vi "EG_G5210 VisaRW.vi"(0 "VISA Rsrc":refnum<visa-resource-name>="GPIB0::12::INSTR", 1 "EOS (Aucun)":string, 5 "ChaineCom":string caption="Chaîne de commande", 6 "Délais (0 ms)":u32, 7 "LockIfc":bool, 9 "Nbcaract":u32=100 caption="Nombre de \ncaractères à lire", 11 "error in (no error)":errorcluster, 12 "Lecture?(T)":bool=TRUE, 13 "Timeout(ms)":u32=2000) -> (4 "VISA Rsrc Out":refnum<visa-resource-name>="GPIB0::12::INSTR", 10 "ChaineRep":string caption="Chaîne de réponse", 14 "Count out":u32=44 caption="Nombre de caractères lus", 15 "error out":errorcluster)   [LabVIEW 2019]
doc: "Ce VI envoie des commande d'écriture et de lecture VISA à l'appareil GPIB. Il permet de ne pas séparer un question de sa réponse. Pour que cela fonctionne toute lecture d'un instrument doit se faire par ce VI."
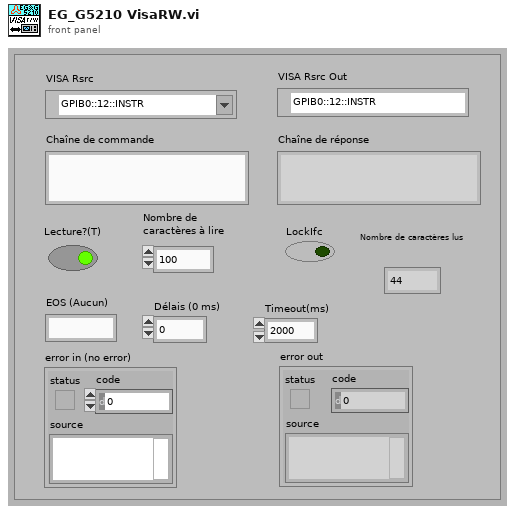
[diagram p1: front panel]
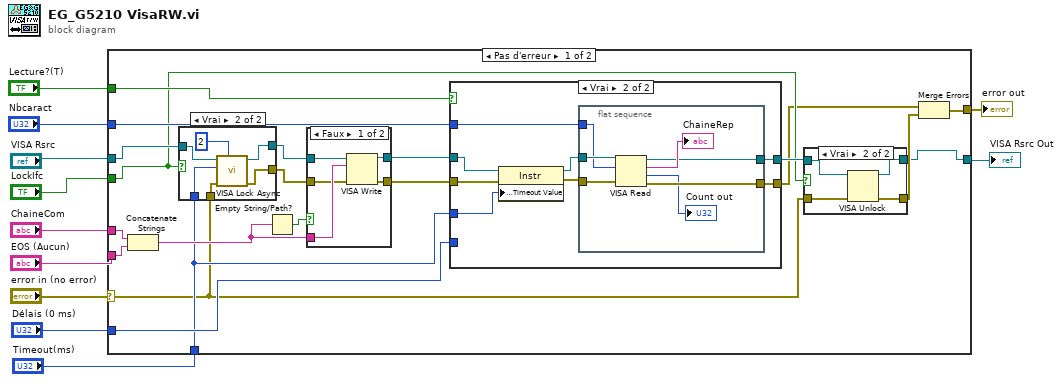
[diagram p0: block diagram]
diagram:
  n1 = case shown="Pas d'erreur" "error in (no error)" {
    selector: "error in (no error)" -> [w16 w71]
    tunnel: "VISA Rsrc" -> [w22 w70]
    tunnel: [w12 w70] -> w3
    tunnel: "ChaineCom" -> [w31 _]
    tunnel: "EOS (Aucun)" -> [w30 _]
    tunnel: "Délais (0 ms)" -> [w27 _]
    tunnel: "Nbcaract" -> [w26 _]
    tunnel: "Lecture?(T)" -> [w25 _]
    tunnel: [w14 w71] -> w5
    tunnel: "Timeout(ms)" -> [w17 _]
    tunnel: "LockIfc" -> [w18 _]
    frame No Error {
      n2 = Concatenate Strings(w31, w30) -> (w23:string)
      n3 = case shown="Vrai" w18 {
        tunnel: [w38 w45] -> w20
        tunnel: w16 -> [w38 w44]
        tunnel: w22 -> [w39 w43]
        tunnel: w17 -> [_ w42]
        tunnel: [w39 w41] -> w21
        frame False {
        }
        frame True {
          n4 = call <vilib>:"VISA Lock Async.vi"("lock type (exclusive: 1)"=u32 2, "error in (no error)"=w44, "timeout (0)"=w42, "VISA resource name"=w43) -> ("error out"=w45:errorcluster, "VISA resource name out"=w41:refnum<visa-resource-name>)  [unwired: 5 in, 1 out]
        }
      }
      n5 = Empty String/Path?(string/path=w23) -> (empty?=w24:bool)
      n6 = case shown="Faux" w24 {
        tunnel: w23 -> [w50 _]
        tunnel: w21 -> [w47 w52]
        tunnel: [w49 w52] -> w29
        tunnel: [w48 w51] -> w28
        tunnel: w20 -> [w46 w51]
        frame False {
          n7 = VISA Write(VISA resource name=w47, write buffer=w50, error in (no error)=w46) -> (VISA resource name out=w49:refnum<visa-resource-name>, error out=w48:errorcluster)  [unwired: 1 out]
        }
        frame True {
        }
      }
      n8 = case shown="Vrai" w25 {
        tunnel: w29 -> [w54 w57]
        tunnel: [w54 w62] -> w19
        tunnel: w28 -> [w53 w59]
        tunnel: [w53 w61] -> w15
        tunnel: w26 -> [_ w60]
        tunnel: w27 -> [_ _]
        tunnel: w17 -> [_ w55]
        frame False {
        }
        frame True {
          n9 = property class="Instr"(reference=w57, error in=w59, "General Settings:Timeout Value"=w55) -> (reference out=w56:refnum<visa-resource-name>, error out=w58:errorcluster)
          n10 = flat-sequence {
            tunnel: [w65] -> w61
            tunnel: [w67] -> w62
            tunnel: w56 -> [w69]
            tunnel: w58 -> [w66]
            tunnel: w60 -> [w63]
            frame #0 {
              n11 = VISA Read(VISA resource name=w69, byte count=w63, error in (no error)=w66) -> (VISA resource name out=w67:refnum<visa-resource-name>, read buffer=→"ChaineRep":string, return count=→"Count out":u32, error out=w65:errorcluster)
            }
          }
        }
      }
      n12 = case shown="Vrai" w18 {
        tunnel: [w32 w37] -> w13
        tunnel: w19 -> [w33 w34]
        tunnel: [w33 w36] -> w12
        tunnel: w16 -> [w32 w35]
        frame False {
        }
        frame True {
          n13 = VISA Unlock(8:w35, 11:w34) -> (0:w37:errorcluster, 3:w36:refnum<visa-resource-name>)
        }
      }
      n14 = Merge Errors(w15, w13) -> (w14:errorcluster)
    }
    frame Error {
    }
  }
  "error out" <- w5
  "VISA Rsrc Out" <- w3
